vi "DSF.Transceiver.UDP.Set Buffer.vi"(10 "buffer":u8[](array[numeric]), 11 "DSF.Transceiver.UDP in":refnum<class "DSF.Transceiver.UDP.lvclass">) -> (3 "DSF.Transceiver.UDP out":refnum<class "DSF.Transceiver.UDP.lvclass">)   [LabVIEW 2017, in "DSF.Transceiver.UDP.lvlib" / "DSF.Transceiver.UDP.lvclass"]
uses:
  DSF.Transceiver.UDP.lvclass
  DSF.Transceiver.UDP.lvclass/DSF.Transceiver.UDP.ctl
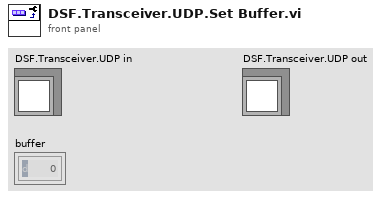
[diagram p1: front panel]
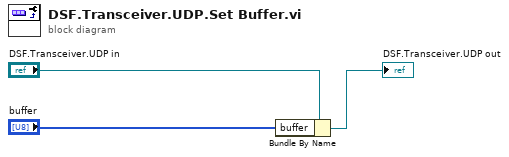
[diagram p0: block diagram]
diagram:
  n1 = Bundle By Name(cluster="DSF.Transceiver.UDP in", "buffer"="buffer") -> (→"DSF.Transceiver.UDP out":refnum<class "DSF.Transceiver.UDP.lvclass">)
